vi "Lab Panel V4.87.vi"() -> ()   [LabVIEW 2013] (continued)
                                n829 = local read "SET LAB04-1"() -> (w1540:T5)
                                n830 = case shown="\"CYCLE TEST\"" w1545 {
                                tunnel: ["L04-1-CHART TEST-" "L04-1-CYCLE TEST-" "L04-1-T-RISE TEST-"] -> w1541
                                frame "CHART TEST", Default {
                                }
                                frame "CYCLE TEST" {
                                }
                                frame "T-RISE TEST" {
                                }
                                }
                                n831 = Unbundle(w1540) -> ("DESCRIPTION"=w1539:string)  [unwired: 4 out]
                                n832 = Concatenate Strings(w1535, "\\", w1533, w1532, w1531, w1532) -> (w1542:string)
                                n833 = String To Path(string=w1542) -> (path=w1544:path)
                                n834 = Concatenate Strings(w1542, w1541, w1539, "-", w1538, ".tdms") -> (w1530:string)
                                n835 = Create Folder(path (use dialog)=w1544) -> (error out=w1543:errorcluster)  [unwired: 2 in, 2 out]
                                n836 = global write "Global 1.vi" "LAB04-1 FILE"(w1530) -> ()
                                n837 = call <vilib>:"Clear Errors.vi"("error in (no error)"=w1543) -> ()  [unwired: 6 in, 1 out]
                              }
                              frame #1 {
                                (unwired) FALSE
                                n838 = String To Path(string=w1554) -> (path=w1550:path)
                                n839 = TDMS Open(6:FALSE, 10:T20."create or replace" ("operation (0:open)"), 11:w1550) -> (0:w1549:errorcluster, 3:→"TDMS LAB04-1":refnum<k34>)  [unwired: 4 in]
                              }
                              frame #2 {
                                n840 = local read "SET LAB04-1"() -> (w1560:T5)
                                n841 = local read "TDMS LAB04-1"() -> (w1571:refnum<k34>)
                                n842 = Build Array("Testers Name", "Description", "Set Test Cycles", "T-Rise minutes", "T-Rise Deg C") -> (w1561:string[])
                                n843 = Unbundle(w1560) -> ("NAME"=w1559:string, "DESCRIPTION"=w1558:string, "CYCLES"=w1557:dbl, "T-RISE mins"=w1556:dbl, "T-RISE deg C"=w1555:dbl)
                                n844 = Number To Decimal String(number=w1557) -> (decimal integer string=w1570:string)  [unwired: 1 in]
                                n845 = Number To Decimal String(number=w1556) -> (decimal integer string=w1569:string)  [unwired: 1 in]
                                n846 = Number To Decimal String(number=w1555) -> (decimal integer string=w1568:string)  [unwired: 1 in]
                                n847 = Build Array(w1559, w1558, w1570, w1569, w1568) -> (w1567:string[])
                                n848 = TDMS Set Properties(5:w1567, 7:w1561, 11:w1571) -> ()  [unwired: 3 in, 4 out]
                              }
                              frame #3 {
                                n849 = local read "DISP LAB04-1"() -> (w1576:T4)
                                n850 = Concatenate Strings("LAB04-1  ", w1575) -> (w1577:string)
                                n851 = Two Button Dialog(message=w1577, 1:w1573, 2:w1574) -> (T button?=w1579:bool)
                                n852 = case shown="True" w1579 {
                                tunnel: w1576 -> [w1586 w1587]
                                tunnel: [w1586 w1587] -> w1583
                                tunnel: [w1585 w1588] -> w1582
                                tunnel: [w1584 w1588] -> w1581
                                frame False {
                                n853 = Unbundle(w1586) -> ("CYCLE"=w1585:dbl, "MINS"=w1584:dbl)  [unwired: 1 out]
                                }
                                frame True {
                                w1588 = 0.0
                                }
                                }
                                n854 = Bundle(cluster=w1583, "CYCLE"=w1582, "MINS"=w1581, "STATUS"="RUN") -> (w1572:T4)
                                n855 = local write "DISP LAB04-1"(w1572) -> ()
                              }
                              frame #4 {
                                n856 = local read "TEMP START LAB04-1"() -> (w1593:cluster{"TL":dbl, "TN":dbl})
                                n857 = Unbundle(w1589) -> ("Tmp Live"=w1591:dbl, "Tmp Neut"=w1590:dbl)  [unwired: 3 out]
                                n858 = Bundle(cluster=w1593, "TL"=w1591, "TN"=w1590) -> (w1592:cluster{"TL":dbl, "TN":dbl})
                                n859 = local write "TEMP START LAB04-1"(w1592) -> ()
                              }
                            }
                          }
                        }
                      }
                    }
                  }
                }
              }
              event "RUN LAB04-2": Value Change {
                n860 = event-data() -> ("NewVal"=w1597:bool)  [unwired: 1 in, 5 out]
                n861 = local write "run lab04-2"(w1597) -> ()
                n862 = case shown="True" w1597 {
                  tunnel: w1603 -> [_ w1640]
                  tunnel: w1602 -> [_ w1639]
                  tunnel: w1600 -> [w1605 w1638]
                  tunnel: w1601 -> [_ w1637]
                  tunnel: w1599 -> [_ w1636]
                  tunnel: [w1604 w1635] -> w1598
                  tunnel: w1596 -> [_ w1634]
                  tunnel: w1595 -> [_ w1633]
                  tunnel: w1594 -> [_ w1632]
                  frame False {
                    # "stop test"
                    n863 = stacked-sequence {
                      tunnel: w1605 -> [w1614 _]
                      tunnel: [w1606 _] -> w1604
                      frame #0 {
                        n864 = local read "DISP LAB04-2"() -> (w1613:T4)
                        n865 = Unbundle(w1613) -> ("CYCLE"=w1611:dbl, "MINS"=w1612:dbl)  [unwired: 1 out]
                        n866 = case shown="\"CYCLE TEST\"" w1614 {
                          tunnel: w1612 -> [_ _ w1621]
                          tunnel: w1611 -> [w1619 w1620 _]
                          tunnel: [w1619 w1620 w1621] -> w1610
                          frame "CHART TEST", Default {
                          }
                          frame "CYCLE TEST" {
                          }
                          frame "T-RISE TEST" {
                          }
                        }
                        n867 = local read "TDMS LAB04-2"() -> (w1618:refnum<k34>)
                        n868 = Build Array("STOPPED") -> (w1615:string[])
                        n869 = Build Array(w1610) -> (w1609:dbl[])
                        n870 = TDMS Write(0:w1618, 5:"TEST RESULT", 7:w1615, 9:w1609) -> (4:w1607:refnum<k34>, 15:w1608:errorcluster)  [unwired: 2 in, 2 out]
                        n871 = TDMS Close(8:w1608, 11:w1607) -> (0:w1606:errorcluster)  [unwired: 1 out]
                      }
                      frame #1 {
                        n872 = local read "DISP LAB04-2"() -> (w1625:T4)
                        n873 = stacked-sequence {
                          tunnel: "LAB04-2" -> [w1627 w1629]
                          frame #0 {
                            n874 = call "sub vi - defrag tdms v1.vi"("panel id"=w1627) -> ("error out"=w1626:errorcluster)  [unwired: 10 in]
                            n875 = local write "data file error"(w1626) -> ()
                          }
                          frame #1 {
                            n876 = call "Save data file to network drive v2.vi"("panel id"=w1629) -> ("network file save error"=w1628:errorcluster)  [unwired: 9 in, 1 out]
                            n877 = local write "RESULT LAB04-2"(FALSE) -> ()
                            n878 = local write "data file error"(w1628) -> ()
                          }
                        }
                        n879 = Bundle(cluster=w1625, "STATUS"="STOP") -> (w1623:T4)  [unwired: 2 in]
                        n880 = local write "DISP LAB04-2"(w1623) -> ()
                      }
                    }
                  }
                  frame True {
                    n881 = local read "SIG LAB04-2"() -> (w1631:T2)
                    n882 = stacked-sequence {
                      seq-local: [w1642 _] -> [_ w1645]
                      tunnel: w1640 -> [_ w1655]
                      tunnel: w1639 -> [_ w1654]
                      tunnel: w1638 -> [_ w1653]
                      tunnel: w1637 -> [_ w1652]
                      tunnel: w1636 -> [_ w1651]
                      tunnel: [_ w1650] -> w1635
                      tunnel: w1634 -> [_ w1649]
                      tunnel: w1633 -> [_ w1648]
                      tunnel: w1632 -> [_ w1647]
                      tunnel: w1631 -> [w1641 w1646]
                      frame #0 {
                        n883 = Unbundle(w1641) -> ("AMPS"=w1644:dbl)  [unwired: 4 out]
                        n884 = call "Check For Amps on v1.vi"("ID"="LAB04-2", "amps"=w1644) -> ("amps"=w1642:bool)  [unwired: 9 in]
                      }
                      frame #1 {
                        n885 = case shown="True" w1645 {
                          tunnel: w1655 -> [_ w1667]
                          tunnel: w1654 -> [_ w1666]
                          tunnel: w1653 -> [_ w1665]
                          tunnel: w1652 -> [_ w1664]
                          tunnel: w1651 -> [_ w1663]
                          tunnel: [errorcluster {"status"=FALSE, "code"=0, "source"=""} ("error out") w1662] -> w1650
                          tunnel: w1649 -> [_ w1661]
                          tunnel: w1648 -> [_ w1660]
                          tunnel: w1647 -> [_ w1659]
                          tunnel: w1646 -> [_ w1658]
                          frame False {
                            w1656 = FALSE
                            n886 = local write "RUN LAB04-2"(w1656) -> ()
                            n887 = local write "run lab04-2"(w1656) -> ()
                          }
                          frame True {
                            n888 = stacked-sequence {
                              seq-local: [w1668 _ _ _ _] -> [_ w1692 _ _ _]
                              tunnel: w1667 -> [w1673 _ _ _ _]
                              tunnel: w1666 -> [w1669 _ _ _ _]
                              tunnel: w1665 -> [w1683 _ _ _ _]
                              tunnel: w1664 -> [w1676 _ _ _ _]
                              tunnel: w1663 -> [w1671 _ _ _ _]
                              tunnel: [_ w1687 _ _ _] -> w1662
                              tunnel: w1661 -> [_ _ _ w1713 _]
                              tunnel: w1660 -> [_ _ _ w1712 _]
                              tunnel: w1659 -> [_ _ _ w1711 _]
                              tunnel: w1658 -> [_ _ _ _ w1727]
                              frame #0 {
                                w1670 = "\\"
                                n889 = local read "SET LAB04-2"() -> (w1678:T5)
                                n890 = case shown="\"CHART TEST\", Default" w1683 {
                                tunnel: ["L04-2-CHART TEST-" "L04-2-CYCLE TEST-" "L04-2-T-RISE TEST-"] -> w1679
                                frame "CHART TEST", Default {
                                }
                                frame "CYCLE TEST" {
                                }
                                frame "T-RISE TEST" {
                                }
                                }
                                n891 = Unbundle(w1678) -> ("DESCRIPTION"=w1677:string)  [unwired: 4 out]
                                n892 = Concatenate Strings(w1673, "\\", w1671, w1670, w1669, w1670) -> (w1680:string)
                                n893 = String To Path(string=w1680) -> (path=w1682:path)
                                n894 = Concatenate Strings(w1680, w1679, w1677, "-", w1676, ".tdms") -> (w1668:string)
                                n895 = Create Folder(path (use dialog)=w1682) -> (error out=w1681:errorcluster)  [unwired: 2 in, 2 out]
                                n896 = global write "Global 1.vi" "LAB04-2 FILE"(w1668) -> ()
                                n897 = call <vilib>:"Clear Errors.vi"("error in (no error)"=w1681) -> ()  [unwired: 6 in, 1 out]
                              }
                              frame #1 {
                                (unwired) FALSE
                                n898 = String To Path(string=w1692) -> (path=w1688:path)
                                n899 = TDMS Open(6:FALSE, 10:T20."create or replace" ("operation (0:open)"), 11:w1688) -> (0:w1687:errorcluster, 3:→"TDMS LAB04-2":refnum<k34>)  [unwired: 4 in]
                              }
                              frame #2 {
                                n900 = local read "SET LAB04-2"() -> (w1698:T5)
                                n901 = local read "TDMS LAB04-2"() -> (w1709:refnum<k34>)
                                n902 = Build Array("Testers Name", "Description", "Set Test Cycles", "T-Rise minutes", "T-Rise Deg C") -> (w1699:string[])
                                n903 = Unbundle(w1698) -> ("NAME"=w1697:string, "DESCRIPTION"=w1696:string, "CYCLES"=w1695:dbl, "T-RISE mins"=w1694:dbl, "T-RISE deg C"=w1693:dbl)
                                n904 = Number To Decimal String(number=w1695) -> (decimal integer string=w1708:string)  [unwired: 1 in]
                                n905 = Number To Decimal String(number=w1694) -> (decimal integer string=w1707:string)  [unwired: 1 in]
                                n906 = Number To Decimal String(number=w1693) -> (decimal integer string=w1706:string)  [unwired: 1 in]
                                n907 = Build Array(w1697, w1696, w1708, w1707, w1706) -> (w1705:string[])
                                n908 = TDMS Set Properties(5:w1705, 7:w1699, 11:w1709) -> ()  [unwired: 3 in, 4 out]
                              }
                              frame #3 {
                                n909 = local read "DISP LAB04-2"() -> (w1714:T4)
                                n910 = Concatenate Strings("LAB04-2 ", w1713) -> (w1715:string)
                                n911 = Two Button Dialog(message=w1715, 1:w1711, 2:w1712) -> (T button?=w1717:bool)
                                n912 = case shown="True" w1717 {
                                tunnel: w1714 -> [w1724 w1725]
                                tunnel: [w1724 w1725] -> w1721
                                tunnel: [w1723 w1726] -> w1720
                                tunnel: [w1722 w1726] -> w1719
                                frame False {
                                n913 = Unbundle(w1724) -> ("CYCLE"=w1723:dbl, "MINS"=w1722:dbl)  [unwired: 1 out]
                                }
                                frame True {
                                w1726 = 0.0
                                }
                                }
                                n914 = Bundle(cluster=w1721, "CYCLE"=w1720, "MINS"=w1719, "STATUS"="RUN") -> (w1710:T4)
                                n915 = local write "DISP LAB04-2"(w1710) -> ()
                              }
                              frame #4 {
                                n916 = local read "TEMP START LAB04-2"() -> (w1731:cluster{"TL":dbl, "TN":dbl})
                                n917 = Unbundle(w1727) -> ("Tmp Live"=w1729:dbl, "Tmp Neut"=w1728:dbl)  [unwired: 3 out]
                                n918 = Bundle(cluster=w1731, "TL"=w1729, "TN"=w1728) -> (w1730:cluster{"TL":dbl, "TN":dbl})
                                n919 = local write "TEMP START LAB04-2"(w1730) -> ()
                              }
                            }
                          }
                        }
                      }
                    }
                  }
                }
              }
              event "RUN LAB05-1": Value Change {
                n920 = event-data() -> ("NewVal"=w1735:bool)  [unwired: 1 in, 5 out]
                n921 = local write "run lab05-1"(w1735) -> ()
                n922 = case shown="True" w1735 {
                  tunnel: w1741 -> [_ w1778]
                  tunnel: w1740 -> [_ w1777]
                  tunnel: w1738 -> [w1743 w1776]
                  tunnel: w1739 -> [_ w1775]
                  tunnel: w1737 -> [_ w1774]
                  tunnel: [w1742 w1773] -> w1736
                  tunnel: w1734 -> [_ w1772]
                  tunnel: w1733 -> [_ w1771]
                  tunnel: w1732 -> [_ w1770]
                  frame False {
                    # "stop test"
                    n923 = stacked-sequence {
                      tunnel: w1743 -> [w1752 _]
                      tunnel: [w1744 _] -> w1742
                      frame #0 {
                        n924 = local read "DISP LAB05-1"() -> (w1751:T4)
                        n925 = Unbundle(w1751) -> ("CYCLE"=w1749:dbl, "MINS"=w1750:dbl)  [unwired: 1 out]
                        n926 = case shown="\"CYCLE TEST\"" w1752 {
                          tunnel: w1750 -> [_ _ w1759]
                          tunnel: w1749 -> [w1757 w1758 _]
                          tunnel: [w1757 w1758 w1759] -> w1748
                          frame "CHART TEST", Default {
                          }
                          frame "CYCLE TEST" {
                          }
                          frame "T-RISE TEST" {
                          }
                        }
                        n927 = local read "TDMS LAB05-1"() -> (w1756:refnum<k34>)
                        n928 = Build Array("STOPPED") -> (w1753:string[])
                        n929 = Build Array(w1748) -> (w1747:dbl[])
                        n930 = TDMS Write(0:w1756, 5:"TEST RESULT", 7:w1753, 9:w1747) -> (4:w1745:refnum<k34>, 15:w1746:errorcluster)  [unwired: 2 in, 2 out]
                        n931 = TDMS Close(8:w1746, 11:w1745) -> (0:w1744:errorcluster)  [unwired: 1 out]
                      }
                      frame #1 {
                        n932 = local read "DISP LAB05-1"() -> (w1763:T4)
                        n933 = stacked-sequence {
                          tunnel: "LAB05-1" -> [w1765 w1767]
                          frame #0 {
                            n934 = call "sub vi - defrag tdms v1.vi"("panel id"=w1765) -> ("error out"=w1764:errorcluster)  [unwired: 10 in]
                            n935 = local write "data file error"(w1764) -> ()
                          }
                          frame #1 {
                            n936 = call "Save data file to network drive v2.vi"("panel id"=w1767) -> ("network file save error"=w1766:errorcluster)  [unwired: 9 in, 1 out]
                            n937 = local write "RESULT LAB05-1"(FALSE) -> ()
                            n938 = local write "data file error"(w1766) -> ()
                          }
                        }
                        n939 = Bundle(cluster=w1763, "STATUS"="STOP") -> (w1761:T4)  [unwired: 2 in]
                        n940 = local write "DISP LAB05-1"(w1761) -> ()
                      }
                    }
                  }
                  frame True {
                    n941 = local read "SIG LAB05-1"() -> (w1769:T2)
                    n942 = stacked-sequence {
                      seq-local: [w1780 _] -> [_ w1783]
                      tunnel: w1778 -> [_ w1793]
                      tunnel: w1777 -> [_ w1792]
                      tunnel: w1776 -> [_ w1791]
                      tunnel: w1775 -> [_ w1790]
                      tunnel: w1774 -> [_ w1789]
                      tunnel: [_ w1788] -> w1773
                      tunnel: w1772 -> [_ w1787]
                      tunnel: w1771 -> [_ w1786]
                      tunnel: w1770 -> [_ w1785]
                      tunnel: w1769 -> [w1779 w1784]
                      frame #0 {
                        n943 = Unbundle(w1779) -> ("AMPS"=w1782:dbl)  [unwired: 4 out]
                        n944 = call "Check For Amps on v1.vi"("ID"="LAB05-1", "amps"=w1782) -> ("amps"=w1780:bool)  [unwired: 9 in]
                      }
                      frame #1 {
                        n945 = case shown="True" w1783 {
                          tunnel: w1793 -> [_ w1805]
                          tunnel: w1792 -> [_ w1804]
                          tunnel: w1791 -> [_ w1803]
                          tunnel: w1790 -> [_ w1802]
                          tunnel: w1789 -> [_ w1801]
                          tunnel: [errorcluster {"status"=FALSE, "code"=0, "source"=""} ("error out") w1800] -> w1788
                          tunnel: w1787 -> [_ w1799]
                          tunnel: w1786 -> [_ w1798]
                          tunnel: w1785 -> [_ w1797]
                          tunnel: w1784 -> [_ w1796]
                          frame False {
                            w1794 = FALSE
                            n946 = local write "RUN LAB05-1"(w1794) -> ()
                            n947 = local write "run lab05-1"(w1794) -> ()
                          }
                          frame True {
                            n948 = stacked-sequence {
                              seq-local: [w1806 _ _ _ _] -> [_ w1830 _ _ _]
                              tunnel: w1805 -> [w1811 _ _ _ _]
                              tunnel: w1804 -> [w1807 _ _ _ _]
                              tunnel: w1803 -> [w1821 _ _ _ _]
                              tunnel: w1802 -> [w1814 _ _ _ _]
                              tunnel: w1801 -> [w1809 _ _ _ _]
                              tunnel: [_ w1825 _ _ _] -> w1800
                              tunnel: w1799 -> [_ _ _ w1850 _]
                              tunnel: w1798 -> [_ _ _ w1849 _]
                              tunnel: w1797 -> [_ _ _ w1848 _]
                              tunnel: w1796 -> [_ _ _ _ w1865]
                              frame #0 {
                                w1808 = "\\"
                                n949 = local read "SET LAB05-1"() -> (w1816:T5)
                                n950 = case shown="\"CYCLE TEST\"" w1821 {
                                tunnel: ["L05-1-CHART TEST-" "L05-1-CYCLE TEST-" "L05-1-T-RISE TEST-"] -> w1817
                                frame "CHART TEST", Default {
                                }
                                frame "CYCLE TEST" {
                                }
                                frame "T-RISE TEST" {
                                }
                                }
                                n951 = Unbundle(w1816) -> ("DESCRIPTION"=w1815:string)  [unwired: 4 out]
                                n952 = Concatenate Strings(w1811, "\\", w1809, w1808, w1807, w1808) -> (w1818:string)
                                n953 = String To Path(string=w1818) -> (path=w1820:path)
                                n954 = Concatenate Strings(w1818, w1817, w1815, "-", w1814, ".tdms") -> (w1806:string)
                                n955 = Create Folder(path (use dialog)=w1820) -> (error out=w1819:errorcluster)  [unwired: 2 in, 2 out]
                                n956 = global write "Global 1.vi" "LAB05-1 FILE"(w1806) -> ()
                                n957 = call <vilib>:"Clear Errors.vi"("error in (no error)"=w1819) -> ()  [unwired: 6 in, 1 out]
                              }
                              frame #1 {
                                (unwired) FALSE
                                n958 = String To Path(string=w1830) -> (path=w1826:path)
                                n959 = TDMS Open(6:FALSE, 10:T20."create or replace" ("operation (0:open)"), 11:w1826) -> (0:w1825:errorcluster, 3:→"TDMS LAB05-1":refnum<k34>)  [unwired: 4 in]
                              }
                              frame #2 {
                                n960 = local read "SET LAB05-1"() -> (w1836:T5)
                                n961 = local read "TDMS LAB05-1"() -> (w1847:refnum<k34>)
                                n962 = Build Array("Testers Name", "Description", "Set Test Cycles", "T-Rise minutes", "T-Rise Deg C") -> (w1837:string[])
                                n963 = Unbundle(w1836) -> ("NAME"=w1835:string, "DESCRIPTION"=w1834:string, "CYCLES"=w1833:dbl, "T-RISE mins"=w1832:dbl, "T-RISE deg C"=w1831:dbl)
                                n964 = Number To Decimal String(number=w1833) -> (decimal integer string=w1846:string)  [unwired: 1 in]
                                n965 = Number To Decimal String(number=w1832) -> (decimal integer string=w1845:string)  [unwired: 1 in]
                                n966 = Number To Decimal String(number=w1831) -> (decimal integer string=w1844:string)  [unwired: 1 in]
                                n967 = Build Array(w1835, w1834, w1846, w1845, w1844) -> (w1843:string[])
                                n968 = TDMS Set Properties(5:w1843, 7:w1837, 11:w1847) -> ()  [unwired: 3 in, 4 out]
                              }
                              frame #3 {
                                n969 = local read "DISP LAB05-1"() -> (w1852:T4)
                                n970 = Concatenate Strings("LAB05-1  ", w1850) -> (w1853:string)
                                n971 = Two Button Dialog(message=w1853, 1:w1848, 2:w1849) -> (T button?=w1855:bool)
                                n972 = case shown="True" w1855 {
                                tunnel: w1852 -> [w1862 w1863]
                                tunnel: [w1862 w1863] -> w1859
                                tunnel: [w1861 w1864] -> w1858
                                tunnel: [w1860 w1864] -> w1857
                                frame False {
                                n973 = Unbundle(w1862) -> ("CYCLE"=w1861:dbl, "MINS"=w1860:dbl)  [unwired: 1 out]
                                }
                                frame True {
                                w1864 = 0.0
                                }
                                }
                                n974 = Bundle(cluster=w1859, "CYCLE"=w1858, "MINS"=w1857, "STATUS"="RUN") -> (w1851:T4)
                                n975 = local write "DISP LAB05-1"(w1851) -> ()
                              }
                              frame #4 {
                                n976 = local read "TEMP START LAB05-1"() -> (w1869:cluster{"TL":dbl, "TN":dbl})
                                n977 = Unbundle(w1865) -> ("Tmp Live"=w1867:dbl, "Tmp Neut"=w1866:dbl)  [unwired: 3 out]
                                n978 = Bundle(cluster=w1869, "TL"=w1867, "TN"=w1866) -> (w1868:cluster{"TL":dbl, "TN":dbl})
                                n979 = local write "TEMP START LAB05-1"(w1868) -> ()
                              }
                            }
                          }
                        }
                      }
                    }
                  }
                }
              }
              event "RUN LAB05-2": Value Change {
                n980 = event-data() -> ("NewVal"=w1874:bool)  [unwired: 1 in, 5 out]
                n981 = local read "SIG LAB05-2"() -> (w1870:T2)
                n982 = case shown="True" w1874 {
                  tunnel: w1880 -> [_ w1917]
                  tunnel: w1879 -> [_ w1916]
                  tunnel: w1877 -> [w1882 w1915]
                  tunnel: w1878 -> [_ w1914]
                  tunnel: w1876 -> [_ w1913]
                  tunnel: [w1881 w1912] -> w1875
                  tunnel: w1873 -> [_ w1911]
                  tunnel: w1872 -> [_ w1910]
                  tunnel: w1871 -> [_ w1909]
                  tunnel: w1870 -> [_ w1908]
                  frame False {
                    # "stop test"
                    n983 = stacked-sequence {
                      tunnel: w1882 -> [w1891 _]
                      tunnel: [w1883 _] -> w1881
                      frame #0 {
                        n984 = local read "DISP LAB05-2"() -> (w1890:T4)
                        n985 = Unbundle(w1890) -> ("CYCLE"=w1888:dbl, "MINS"=w1889:dbl)  [unwired: 1 out]
                        n986 = case shown="\"CYCLE TEST\"" w1891 {
                          tunnel: w1889 -> [_ _ w1898]
                          tunnel: w1888 -> [w1896 w1897 _]
                          tunnel: [w1896 w1897 w1898] -> w1887
                          frame "CHART TEST", Default {
                          }
                          frame "CYCLE TEST" {
                          }
                          frame "T-RISE TEST" {
                          }
                        }
                        n987 = local read "TDMS LAB05-2"() -> (w1895:refnum<k34>)
                        n988 = Build Array("STOPPED") -> (w1892:string[])
                        n989 = Build Array(w1887) -> (w1886:dbl[])
                        n990 = TDMS Write(0:w1895, 5:"TEST RESULT", 7:w1892, 9:w1886) -> (4:w1884:refnum<k34>, 15:w1885:errorcluster)  [unwired: 2 in, 2 out]
                        n991 = TDMS Close(8:w1885, 11:w1884) -> (0:w1883:errorcluster)  [unwired: 1 out]
                      }
                      frame #1 {
                        n992 = local read "DISP LAB05-2"() -> (w1902:T4)
                        n993 = stacked-sequence {
                          tunnel: "LAB05-2" -> [w1904 w1906]
                          frame #0 {
                            n994 = call "sub vi - defrag tdms v1.vi"("panel id"=w1904) -> ("error out"=w1903:errorcluster)  [unwired: 10 in]
                            n995 = local write "data file error"(w1903) -> ()
                          }
                          frame #1 {
                            n996 = local write "RESULT LAB05-2"(FALSE) -> ()
                            n997 = call "Save data file to network drive v2.vi"("panel id"=w1906) -> ("network file save error"=w1905:errorcluster)  [unwired: 9 in, 1 out]
                            n998 = local write "data file error"(w1905) -> ()
                          }
                        }
                        n999 = Bundle(cluster=w1902, "STATUS"="STOP") -> (w1900:T4)  [unwired: 2 in]
                        n1000 = local write "DISP LAB05-2"(w1900) -> ()
                      }
                    }
                  }
                  frame True {
                    n1001 = stacked-sequence {
                      seq-local: [w1919 _] -> [_ w1922]
                      tunnel: w1917 -> [_ w1932]
                      tunnel: w1916 -> [_ w1931]
                      tunnel: w1915 -> [_ w1930]
                      tunnel: w1914 -> [_ w1929]
                      tunnel: w1913 -> [_ w1928]
                      tunnel: [_ w1927] -> w1912
                      tunnel: w1911 -> [_ w1926]
                      tunnel: w1910 -> [_ w1925]
                      tunnel: w1909 -> [_ w1924]
                      tunnel: w1908 -> [w1918 w1923]
                      frame #0 {
                        n1002 = Unbundle(w1918) -> ("AMPS"=w1921:dbl)  [unwired: 4 out]
                        n1003 = call "Check For Amps on v1.vi"("ID"="LAB05-2", "amps"=w1921) -> ("amps"=w1919:bool)  [unwired: 9 in]
                      }
                      frame #1 {
                        n1004 = case shown="True" w1922 {
                          tunnel: w1932 -> [_ w1944]
                          tunnel: w1931 -> [_ w1943]
                          tunnel: w1930 -> [_ w1942]
                          tunnel: w1929 -> [_ w1941]
                          tunnel: w1928 -> [_ w1940]
                          tunnel: [errorcluster {"status"=FALSE, "code"=0, "source"=""} ("error out") w1939] -> w1927
                          tunnel: w1926 -> [_ w1938]
                          tunnel: w1925 -> [_ w1937]
                          tunnel: w1924 -> [_ w1936]
                          tunnel: w1923 -> [_ w1935]
                          frame False {
                            w1933 = FALSE
                            n1005 = local write "RUN LAB05-2"(w1933) -> ()
                            n1006 = local write "run lab05-2"(w1933) -> ()
                          }
                          frame True {
                            n1007 = stacked-sequence {
                              seq-local: [w1945 _ _ _ _] -> [_ w1969 _ _ _]
                              tunnel: w1944 -> [w1950 _ _ _ _]
                              tunnel: w1943 -> [w1946 _ _ _ _]
                              tunnel: w1942 -> [w1960 _ _ _ _]
                              tunnel: w1941 -> [w1953 _ _ _ _]
                              tunnel: w1940 -> [w1948 _ _ _ _]
                              tunnel: [_ w1964 _ _ _] -> w1939
                              tunnel: w1938 -> [_ _ _ w1989 _]
                              tunnel: w1937 -> [_ _ _ w1988 _]
                              tunnel: w1936 -> [_ _ _ w1987 _]
                              tunnel: w1935 -> [_ _ _ _ w2004]
                              frame #0 {
                                w1947 = "\\"
                                n1008 = local read "SET LAB05-2"() -> (w1955:T5)
                                n1009 = case shown="\"CYCLE TEST\"" w1960 {
                                tunnel: ["L05-2-CHART TEST-" "L05-2-CYCLE TEST-" "L05-2-T-RISE TEST-"] -> w1956
                                frame "CHART TEST", Default {
                                }
                                frame "CYCLE TEST" {
                                }
                                frame "T-RISE TEST" {
                                }
                                }
                                n1010 = Unbundle(w1955) -> ("DESCRIPTION"=w1954:string)  [unwired: 4 out]
                                n1011 = Concatenate Strings(w1950, "\\", w1948, w1947, w1946, w1947) -> (w1957:string)
                                n1012 = String To Path(string=w1957) -> (path=w1959:path)
                                n1013 = Concatenate Strings(w1957, w1956, w1954, "-", w1953, ".tdms") -> (w1945:string)
                                n1014 = Create Folder(path (use dialog)=w1959) -> (error out=w1958:errorcluster)  [unwired: 2 in, 2 out]
                                n1015 = global write "Global 1.vi" "LAB05-2 FILE"(w1945) -> ()
                                n1016 = call <vilib>:"Clear Errors.vi"("error in (no error)"=w1958) -> ()  [unwired: 6 in, 1 out]
                              }
                              frame #1 {
                                (unwired) FALSE
                                n1017 = String To Path(string=w1969) -> (path=w1965:path)
                                n1018 = TDMS Open(6:FALSE, 10:T20."create or replace" ("operation (0:open)"), 11:w1965) -> (0:w1964:errorcluster, 3:→"TDMS LAB05-2":refnum<k34>)  [unwired: 4 in]
                              }
                              frame #2 {
                                n1019 = local read "SET LAB05-2"() -> (w1975:T5)
                                n1020 = local read "TDMS LAB05-2"() -> (w1986:refnum<k34>)
                                n1021 = Build Array("Testers Name", "Description", "Set Test Cycles", "T-Rise minutes", "T-Rise Deg C") -> (w1976:string[])
                                n1022 = Unbundle(w1975) -> ("NAME"=w1974:string, "DESCRIPTION"=w1973:string, "CYCLES"=w1972:dbl, "T-RISE mins"=w1971:dbl, "T-RISE deg C"=w1970:dbl)
                                n1023 = Number To Decimal String(number=w1972) -> (decimal integer string=w1985:string)  [unwired: 1 in]
                                n1024 = Number To Decimal String(number=w1971) -> (decimal integer string=w1984:string)  [unwired: 1 in]
                                n1025 = Number To Decimal String(number=w1970) -> (decimal integer string=w1983:string)  [unwired: 1 in]
                                n1026 = Build Array(w1974, w1973, w1985, w1984, w1983) -> (w1982:string[])
                                n1027 = TDMS Set Properties(5:w1982, 7:w1976, 11:w1986) -> ()  [unwired: 3 in, 4 out]
                              }
                              frame #3 {
                                n1028 = local read "DISP LAB05-2"() -> (w1991:T4)
                                n1029 = Concatenate Strings("LAB05-2  ", w1989) -> (w1992:string)
                                n1030 = Two Button Dialog(message=w1992, 1:w1987, 2:w1988) -> (T button?=w1994:bool)
                                n1031 = case shown="True" w1994 {
                                tunnel: w1991 -> [w2001 w2002]
                                tunnel: [w2001 w2002] -> w1998
                                tunnel: [w2000 w2003] -> w1997
                                tunnel: [w1999 w2003] -> w1996
                                frame False {
                                n1032 = Unbundle(w2001) -> ("CYCLE"=w2000:dbl, "MINS"=w1999:dbl)  [unwired: 1 out]
                                }
                                frame True {
                                w2003 = 0.0
                                }
                                }
                                n1033 = Bundle(cluster=w1998, "CYCLE"=w1997, "MINS"=w1996, "STATUS"="RUN") -> (w1990:T4)
                                n1034 = local write "DISP LAB05-2"(w1990) -> ()
                              }
                              frame #4 {
                                n1035 = local read "TEMP START LAB05-2"() -> (w2008:cluster{"TL":dbl, "TN":dbl})
                                n1036 = Unbundle(w2004) -> ("Tmp Live"=w2006:dbl, "Tmp Neut"=w2005:dbl)  [unwired: 3 out]
                                n1037 = Bundle(cluster=w2008, "TL"=w2006, "TN"=w2005) -> (w2007:cluster{"TL":dbl, "TN":dbl})
                                n1038 = local write "TEMP START LAB05-2"(w2007) -> ()
                              }
                            }
                          }
                        }
                      }
                    }
                  }
                }
                n1039 = local write "run lab05-2"(w1874) -> ()
              }
            }
            n1040 = local write "data file error"(w597) -> ()
          }
          frame #4 {
            # "check if test cycles reached for cycle tests, if so then test pass"
            n1041 = stacked-sequence {
              tunnel: w2028 -> [_ _ _ _ _ _ _ _ _ _]
              tunnel: w2027 -> [_ _ _ _ _ _ _ _ _ _]
              tunnel: w2026 -> [_ _ _ _ _ _ _ _ _ _]
              tunnel: w2025 -> [_ _ _ _ _ _ _ _ _ _]
              tunnel: w2024 -> [_ _ _ _ _ _ _ _ _ _]
              tunnel: w2023 -> [_ _ _ _ _ _ _ _ _ _]
              tunnel: w2022 -> [_ _ _ _ _ _ _ _ _ _]
              tunnel: w2021 -> [_ _ _ _ _ _ _ _ _ _]
              tunnel: w2020 -> [_ _ _ _ _ _ _ _ _ _]
              tunnel: w2019 -> [_ _ _ _ _ _ _ _ _ _]
              tunnel: w2018 -> [w2034 _ _ _ _ _ _ _ _ _]
              tunnel: w2017 -> [_ w2069 _ _ _ _ _ _ _ _]
              tunnel: w2016 -> [_ _ w2109 _ _ _ _ _ _ _]
              tunnel: w2015 -> [_ _ _ w2149 _ _ _ _ _ _]
              tunnel: w2014 -> [_ _ _ _ w2189 _ _ _ _ _]
              tunnel: w2013 -> [_ _ _ _ _ w2229 _ _ _ _]
              tunnel: w2012 -> [_ _ _ _ _ _ w2269 _ _ _]
              tunnel: w2011 -> [_ _ _ _ _ _ _ w2309 _ _]
              tunnel: w2010 -> [_ _ _ _ _ _ _ _ w2349 _]
              tunnel: w2009 -> [_ _ _ _ _ _ _ _ _ w2389]
              frame #0 {
                # "LAB01-1"
                n1042 = Less?(x=w2034, y=2) -> (x < y?=w2032:bool)
                n1043 = local read "DISP LAB01-1"() -> (w2035:T4)
                n1044 = Unbundle(w2035) -> ("STATUS"=w2029:string)  [unwired: 2 out]
                n1045 = Equal?(x=w2029, y="RUN") -> (x = y?=w2031:bool)
                n1046 = And(x=w2031, y=w2032) -> (x .and. y?=w2030:bool)
                n1047 = case shown="True" w2030 {
                  tunnel: w2035 -> [_ w2040]
                  tunnel: w2034 -> [_ w2044]
                  frame False {
                  }
                  frame True {
                    n1048 = local read "SET LAB01-1"() -> (w2046:T5)
                    n1049 = local read "TDMS LAB01-1"() -> (w2039:refnum<k34>)
                    n1050 = Unbundle(w2046) -> ("CYCLES"=w2037:dbl, "T-RISE mins"=w2043:dbl)  [unwired: 3 out]
                    n1051 = case shown="\"CYCLE TEST\"" w2044 {
                      tunnel: w2043 -> [_ _ w2053]
                      tunnel: [w2048 w2050 w2053] -> w2042
                      tunnel: w2037 -> [w2048 w2050 _]
                      tunnel: ["CHART PASS" "CYCLE PASS" "T-RISE PASS"] -> w2041
                      frame "CHART TEST", Default {
                      }
                      frame "CYCLE TEST" {
                      }
                      frame "T-RISE TEST" {
                      }
                    }
                    n1052 = Unbundle(w2040) -> ("CYCLE"=w2045:dbl)  [unwired: 2 out]
                    n1053 = Increment(x=w2037) -> (x+1=w2038:dbl)
                    n1054 = Greater Or Equal?(x=w2045, y=w2038) -> (x >= y?=w2047:bool)
                    n1055 = case shown="True" w2047 {
                      tunnel: w2042 -> [w2057 _]
                      tunnel: w2041 -> [w2056 _]
                      tunnel: w2040 -> [w2055 _]
                      tunnel: w2039 -> [w2054 _]
                      frame True {
                        n1056 = stacked-sequence {
                          tunnel: w2057 -> [w2061 _]
                          tunnel: w2056 -> [w2059 w2065]
                          tunnel: w2055 -> [_ w2068]
                          tunnel: w2054 -> [w2058 _]
                          frame #0 {
                            n1057 = Build Array(w2059) -> (w2062:string[])
                            n1058 = Build Array(w2061) -> (w2060:dbl[])
                            n1059 = TDMS Write(0:w2058, 5:"TEST PASS", 7:w2062, 9:w2060) -> (15:w2064:errorcluster)  [unwired: 2 in, 3 out]
                            n1060 = local write "data file error"(w2064) -> ()
                          }
                          frame #1 {
                            n1061 = Bundle(cluster=w2068, "STATUS"=w2065) -> (w2066:T4)  [unwired: 2 in]
                            n1062 = local write "RESULT LAB01-1"(TRUE) -> ()
                            n1063 = local write "DISP LAB01-1"(w2066) -> ()
                          }
                        }
                      }
                      frame False {
                      }
                    }
                  }
                }
              }
              frame #1 {
                # "LAB01-2"
                n1064 = Less?(x=w2069, y=2) -> (x < y?=w2072:bool)
                n1065 = local read "DISP LAB01-2"() -> (w2074:T4)
                n1066 = Unbundle(w2074) -> ("STATUS"=w2075:string)  [unwired: 2 out]
                n1067 = Equal?(x=w2075, y="RUN") -> (x = y?=w2071:bool)
                n1068 = And(x=w2071, y=w2072) -> (x .and. y?=w2070:bool)
                n1069 = case shown="True" w2070 {
                  tunnel: w2074 -> [_ w2080]
                  tunnel: w2069 -> [_ w2084]
                  frame False {
                  }
                  frame True {
                    n1070 = local read "SET LAB01-2"() -> (w2086:T5)
                    n1071 = local read "TDMS LAB01-2"() -> (w2079:refnum<k34>)
                    n1072 = Unbundle(w2086) -> ("CYCLES"=w2077:dbl, "T-RISE mins"=w2083:dbl)  [unwired: 3 out]
                    n1073 = case shown="\"T-RISE TEST\"" w2084 {
                      tunnel: w2083 -> [_ _ w2093]
                      tunnel: [w2088 w2090 w2093] -> w2082
                      tunnel: w2077 -> [w2088 w2090 _]
                      tunnel: ["CHART PASS" "CYCLE PASS" "T-RISE PASS"] -> w2081
                      frame "CHART TEST", Default {
                      }
                      frame "CYCLE TEST" {
                      }
                      frame "T-RISE TEST" {
                      }
                    }
                    n1074 = Unbundle(w2080) -> ("CYCLE"=w2085:dbl)  [unwired: 2 out]
                    n1075 = Increment(x=w2077) -> (x+1=w2078:dbl)
                    n1076 = Greater Or Equal?(x=w2085, y=w2078) -> (x >= y?=w2087:bool)
                    n1077 = case shown="True" w2087 {
                      tunnel: w2082 -> [w2097 _]
                      tunnel: w2081 -> [w2096 _]
                      tunnel: w2080 -> [w2095 _]
                      tunnel: w2079 -> [w2094 _]
                      frame True {
                        n1078 = stacked-sequence {
                          tunnel: w2097 -> [w2101 _]
                          tunnel: w2096 -> [w2099 w2105]
                          tunnel: w2095 -> [_ w2108]
                          tunnel: w2094 -> [w2098 _]
                          frame #0 {
                            n1079 = Build Array(w2099) -> (w2102:string[])
                            n1080 = Build Array(w2101) -> (w2100:dbl[])
                            n1081 = TDMS Write(0:w2098, 5:"TEST PASS", 7:w2102, 9:w2100) -> (15:w2104:errorcluster)  [unwired: 2 in, 3 out]
                            n1082 = local write "data file error"(w2104) -> ()
                          }
                          frame #1 {
                            n1083 = Bundle(cluster=w2108, "STATUS"=w2105) -> (w2106:T4)  [unwired: 2 in]
                            n1084 = local write "RESULT LAB01-2"(TRUE) -> ()
                            n1085 = local write "DISP LAB01-2"(w2106) -> ()
                          }
                        }
                      }
                      frame False {
                      }
                    }
                  }
                }
              }
              frame #2 {
                # "LAB02-1"
                n1086 = Less?(x=w2109, y=2) -> (x < y?=w2112:bool)
                n1087 = local read "DISP LAB02-1"() -> (w2114:T4)
                n1088 = Unbundle(w2114) -> ("STATUS"=w2115:string)  [unwired: 2 out]
                n1089 = Equal?(x=w2115, y="RUN") -> (x = y?=w2111:bool)
                n1090 = And(x=w2111, y=w2112) -> (x .and. y?=w2110:bool)
                n1091 = case shown="True" w2110 {
                  tunnel: w2114 -> [_ w2120]
                  tunnel: w2109 -> [_ w2124]
                  frame False {
                  }
                  frame True {
                    n1092 = local read "SET LAB02-1"() -> (w2126:T5)
                    n1093 = local read "TDMS LAB02-1"() -> (w2119:refnum<k34>)
                    n1094 = Unbundle(w2120) -> ("CYCLE"=w2125:dbl)  [unwired: 2 out]
                    n1095 = Unbundle(w2126) -> ("CYCLES"=w2117:dbl, "T-RISE mins"=w2123:dbl)  [unwired: 3 out]
                    n1096 = case shown="\"T-RISE TEST\"" w2124 {
                      tunnel: w2123 -> [_ _ w2133]
                      tunnel: [w2128 w2130 w2133] -> w2122
                      tunnel: w2117 -> [w2128 w2130 _]
                      tunnel: ["CHART PASS" "CYCLE PASS" "T-RISE PASS"] -> w2121
                      frame "CHART TEST", Default {
                      }
                      frame "CYCLE TEST" {
                      }
                      frame "T-RISE TEST" {
                      }
                    }
                    n1097 = Increment(x=w2117) -> (x+1=w2118:dbl)
                    n1098 = Greater Or Equal?(x=w2125, y=w2118) -> (x >= y?=w2127:bool)
                    n1099 = case shown="True" w2127 {
                      tunnel: w2122 -> [w2137 _]
                      tunnel: w2121 -> [w2136 _]
                      tunnel: w2120 -> [w2135 _]
                      tunnel: w2119 -> [w2134 _]
                      frame True {
                        n1100 = stacked-sequence {
                          tunnel: w2137 -> [w2141 _]
                          tunnel: w2136 -> [w2139 w2145]
                          tunnel: w2135 -> [_ w2148]
                          tunnel: w2134 -> [w2138 _]
                          frame #0 {
                            n1101 = Build Array(w2139) -> (w2142:string[])
                            n1102 = Build Array(w2141) -> (w2140:dbl[])
                            n1103 = TDMS Write(0:w2138, 5:"TEST PASS", 7:w2142, 9:w2140) -> (15:w2144:errorcluster)  [unwired: 2 in, 3 out]
                            n1104 = local write "data file error"(w2144) -> ()
                          }
                          frame #1 {
                            n1105 = Bundle(cluster=w2148, "STATUS"=w2145) -> (w2146:T4)  [unwired: 2 in]
                            n1106 = local write "RESULT LAB02-1"(TRUE) -> ()
                            n1107 = local write "DISP LAB02-1"(w2146) -> ()
                          }
                        }
                      }
                      frame False {
                      }
                    }
                  }
                }
              }
              frame #3 {
                # "LAB02-2"
                n1108 = Less?(x=w2149, y=2) -> (x < y?=w2152:bool)
                n1109 = local read "DISP LAB02-2"() -> (w2154:T4)
                n1110 = Unbundle(w2154) -> ("STATUS"=w2155:string)  [unwired: 2 out]
                n1111 = Equal?(x=w2155, y="RUN") -> (x = y?=w2151:bool)
                n1112 = And(x=w2151, y=w2152) -> (x .and. y?=w2150:bool)
                n1113 = case shown="True" w2150 {
                  tunnel: w2154 -> [_ w2160]
                  tunnel: w2149 -> [_ w2164]
                  frame False {
                  }
                  frame True {
                    n1114 = local read "SET LAB02-2"() -> (w2166:T5)
                    n1115 = local read "TDMS LAB02-2"() -> (w2159:refnum<k34>)
                    n1116 = Unbundle(w2160) -> ("CYCLE"=w2165:dbl)  [unwired: 2 out]
                    n1117 = Unbundle(w2166) -> ("CYCLES"=w2157:dbl, "T-RISE mins"=w2163:dbl)  [unwired: 3 out]
                    n1118 = case shown="\"T-RISE TEST\"" w2164 {
                      tunnel: w2163 -> [_ _ w2173]
                      tunnel: [w2168 w2170 w2173] -> w2162
                      tunnel: w2157 -> [w2168 w2170 _]
                      tunnel: ["CHART PASS" "CYCLE PASS" "T-RISE PASS"] -> w2161
                      frame "CHART TEST", Default {
                      }
